vi "Update JSON Config.vi"(8 "error in (no error)":errorcluster, 10 "Parameter and Value":string="SETCONF=SMUResourceName[[CONFPARAM]]=SMU", 11 "JSON Configuration File (.json)":path=path "C:/Users/chericks/Desktop/JSONtest/labview-grpc-query-server/jsontestfile2.json") -> (0 "error out":errorcluster)   [LabVIEW 2019]
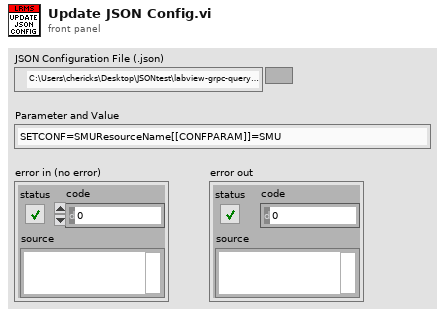
[diagram p1: front panel]
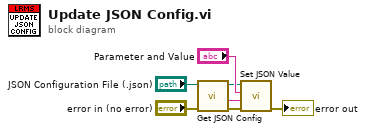
[diagram p0: block diagram]
diagram:
  n1 = call "Get JSON Config.vi"("error in (no error)"="error in (no error)", "JSON Configuration File (.json)"="JSON Configuration File (.json)") -> ("error out"=w3:errorcluster, "File Contents"=w4:string, "JSON Configuration File (.json) out"=w2:path)  [unwired: 6 in, 1 out]
  n2 = call "Set JSON Value.vi"("error in (no error)"=w3, "File Contents"=w4, "Parameter and Value"="Parameter and Value", "JSON Configuration File (.json)"=w2) -> ("error out"=→"error out":errorcluster)  [unwired: 7 in]
